vi "Get Display Text.vi"(8 "error in (no error)":errorcluster, 11 "Data Item in":refnum<class "Data Item.lvclass">) -> (0 "error out":errorcluster, 1 "Detail Text":string, 2 "Display Name":string, 3 "Data Item out":refnum<class "Data Item.lvclass">)   [LabVIEW 2018, in "VILab.lvlib" / "Data Item.lvclass"]
uses:
  Data Item.lvclass
  Data Item.lvclass/Data Item.ctl
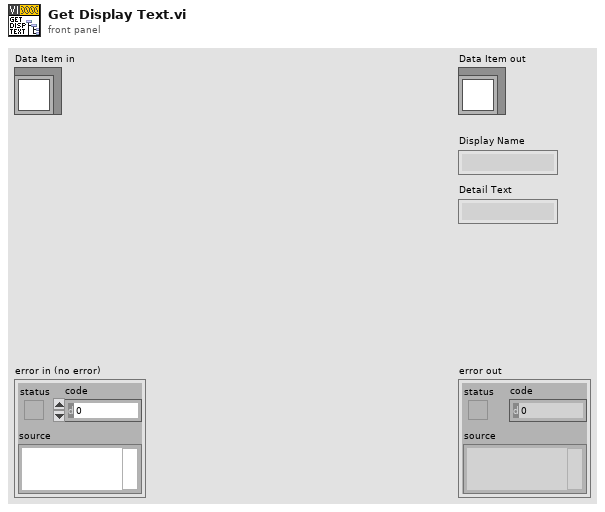
[diagram p1: front panel]
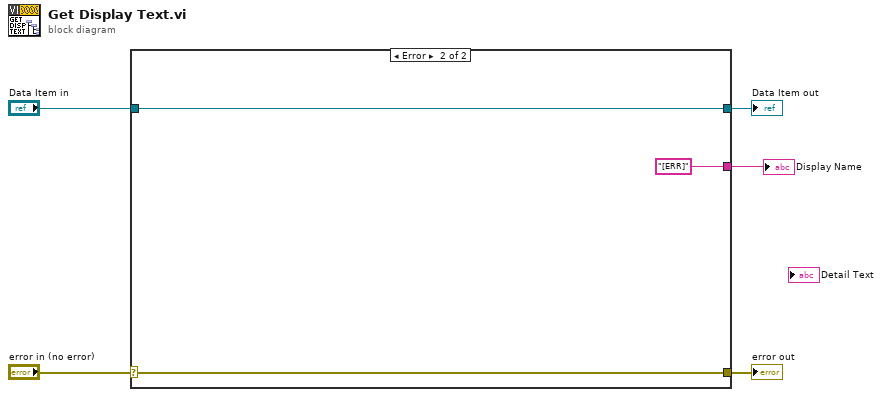
[diagram p0: block diagram]
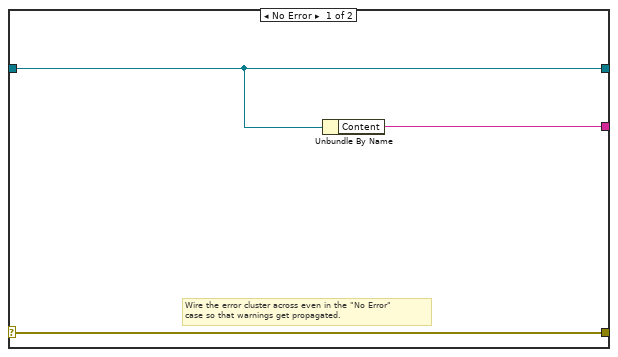
[diagram p2: hidden frame]
diagram:
  n1 = case shown="Error" "error in (no error)" {
    selector: "error in (no error)" -> [w8 w11]
    tunnel: [w8 w11] -> w4
    tunnel: [w7 w10] -> w2
    tunnel: "Data Item in" -> [w7 w10]
    tunnel: [w6 "[ERR]"] -> w1
    frame No Error {
      # "Wire the error cluster across even in the \"No Error\"\ncase so that warnings get propagated."
      n2 = Unbundle By Name(w7) -> ("Content"=w6:string)
    }
    frame Error {
    }
  }
  "error out" <- w4
  "Data Item out" <- w2
  "Display Name" <- w1
